vi "Failure Message.vi"() -> ()   [LabVIEW 2017, in "Assertions.Tests.lvlib" / "Assert String Ends With.lvlib"]
uses:
  Assert String Ends With.lvlib
  src/Transparent Assertions/Assertions/Assertions.lvlib
panel:
  out "error out":errorcluster
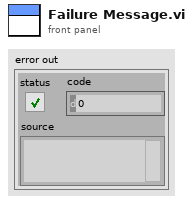
[diagram p1: front panel]
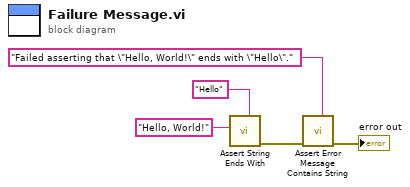
[diagram p0: block diagram]
diagram:
  n1 = call "Assert String Ends With.vi"("Suffix"="Hello", "String"="Hello, World!") -> ("error out"=w3:errorcluster)  [unwired: 9 in]
  n2 = call "Assert Error Message Contains String.vi"("Expected"="Failed asserting that \"Hello, World!\" ends with \"Hello\".", "error in (no error)"=w3) -> ("error out"=→"error out":errorcluster)  [unwired: 9 in]
